vi "Custom Error Dialog.vi"(8 "error in (no error)":errorcluster, 10 "Step Info":string, 11 "Sequence Context":refnum<k7>) -> (3 "Terminate?":bool)   [LabVIEW 2013]
doc: "Error dialog to handle simulation driver errors and provide troubleshooting information. This dialog is intended to replace the default error dialog for codes -10 to 0."
panel:
  out "Step Info":string
  in  "Terminate":bool
  in  "Ignore":bool
  out "Troubleshooting Info":string
  out "Error Details":string
  out "Error Code":i32
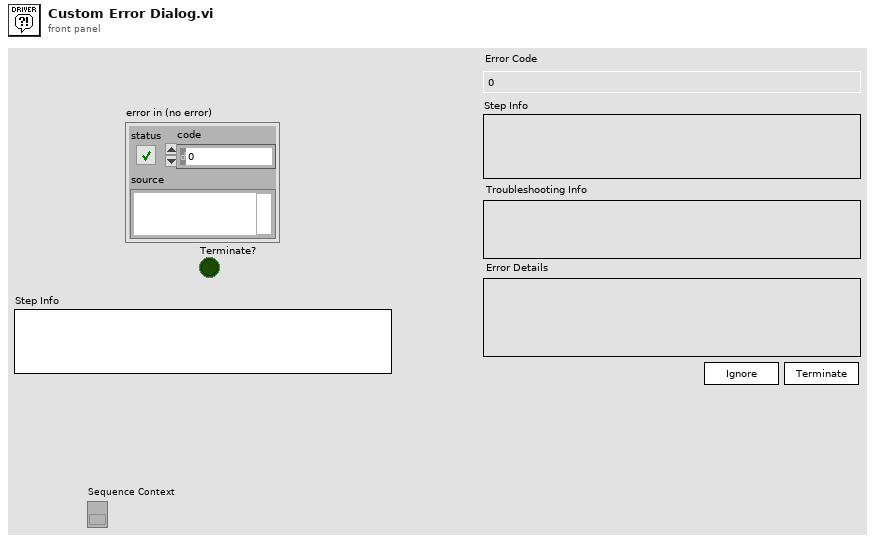
[diagram p1: front panel]
types:
  T1 = cluster{"code":i32, "troubleshooting information":string}[]
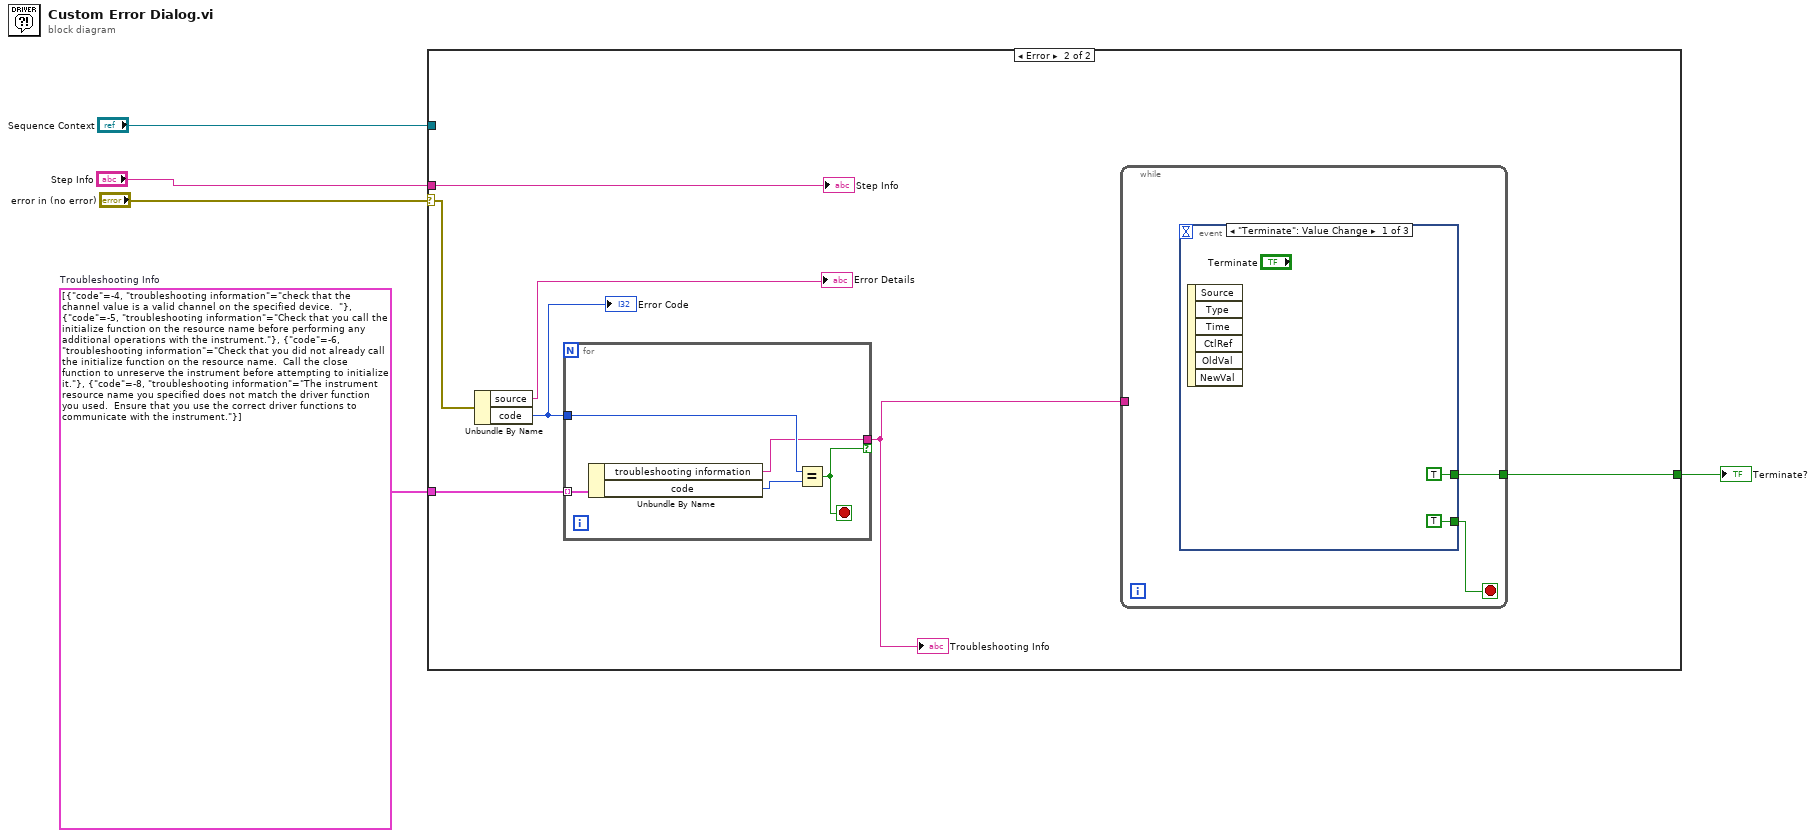
[diagram p0: block diagram]
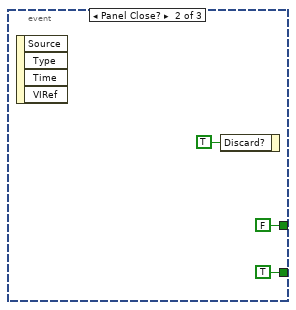
[diagram p3: hidden frame]
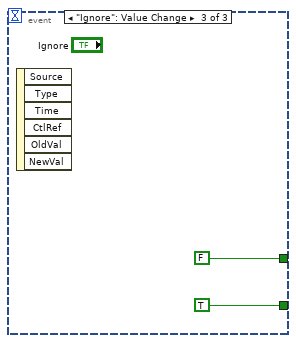
[diagram p4: hidden frame]
diagram:
  w4 = T1 [{"code"=-4, "troubleshooting information"="check that the channel value is a valid channel on the specified device.  "}, {"code"=-5, "troubleshooting information"="Check that you call the initialize function on the resource name before performing any additional operations with the instrument."}, {"code"=-6, "troubleshooting information"="Check that you did not already call the initialize function on the resource name.  Call the close function to unreserve the instrument before attempting to initialize it."}, {"code"=-8, "troubleshooting information"="The instrument resource name you specified does not match the driver function you used.  Ensure that you use the correct driver functions to communicate with the instrument."}]  # Troubleshooting Info
  n1 = case shown="Error" "error in (no error)" {
    selector: "error in (no error)" -> [_ w8]
    tunnel: w4 -> [_ w12]
    tunnel: "Step Info" -> [_ w10]
    tunnel: [_ w6] -> w2
    tunnel: "Sequence Context" -> [_ _]
    frame No Error {
    }
    frame Error {
      n2 = Unbundle By Name(w8) -> ("source"=→"Error Details":string, "code"=w11:i32)
      "Error Code" <- w11
      n3 = for {
        tunnel: w12 -> [w26] mode=indexing
        tunnel: w11 -> [w24]
        tunnel: [w23] -> w7 if=w22
        stop <- w22 stop-if-true
        n4 = Unbundle By Name(w26) -> ("troubleshooting information"=w23:string, "code"=w25:i32)
        n5 = Equal?(x=w24, y=w25) -> (x = y?=w22:bool)
      }
      "Troubleshooting Info" <- w7
      n6 = while {
        tunnel: [w13] -> w6
        tunnel: w7 -> [_]
        stop <- w14 stop-if-true
        n7 = event shown="[0] \"Terminate\": Value Change" {
          selector: _ -> [_ _ _]
          dyn-events: _ -> [_ _ _]
          timeout: _ -> [_ _ _]
          tunnel: [TRUE TRUE TRUE] -> w14
          tunnel: [TRUE FALSE FALSE] -> w13
          event "Terminate": Value Change {
            n8 = event-data() -> ()  [unwired: 1 in, 6 out]
          }
          event Panel Close? {
            n9 = event-data() -> ()  [unwired: 1 in, 4 out]
            n10 = event-data("Discard?"=TRUE) -> ()  [unwired: 1 in, 1 out]
          }
          event "Ignore": Value Change {
            n11 = event-data() -> ()  [unwired: 1 in, 6 out]
          }
        }
      }
      "Step Info" <- w10
    }
  }
  "Terminate?" <- w2
